vi "Memory.Pointer.Errors.vi"   [LabVIEW 2016, in "Memory Manager.lvlib" / "Memory.Pointer.lvclass"]
uses:
  Memory.Pointer.lvclass
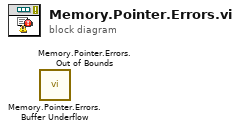
[diagram p0: block diagram]
diagram:
  n1 = call "Memory.Pointer.Errors.Buffer Underflow.vi"() -> ()  [unwired: 10 in, 2 out]
  n2 = call "Memory.Pointer.Errors.Out of Bounds.vi"() -> ()  [unwired: 10 in, 2 out]
